vi "sgl-u8s.vi"(1 "输入sgl":sgl=100.0, 4 "精度":sgl) -> (8 "u8s":u8[](array[numeric]))   [LabVIEW 2012]
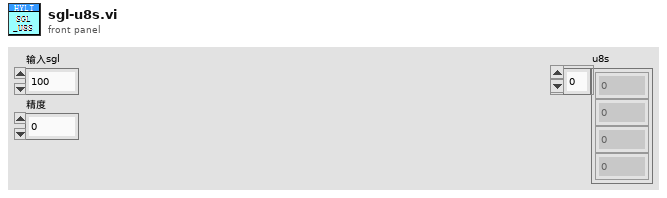
[diagram p1: front panel]
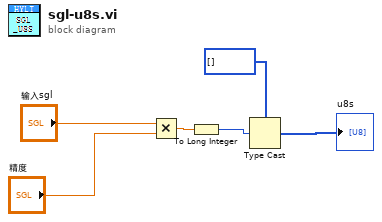
[diagram p0: block diagram]
diagram:
  n1 = Multiply(x="输入sgl", y="精度") -> (x*y=w6:sgl)
  n2 = To Long Integer(number=w6) -> (32bit integer=w4:i32)
  n3 = Type Cast(type=u8[] [], x=w4) -> (*(type *) &x=→"u8s":u8[])
